vi "纳清叶绿素a电极校准.vi"() -> ()   [LabVIEW 2016, in "斯坦道多参数.lvlib"]
uses:
  <vilib>/Utility/miscctls.llb/LVPointTypeDef.ctl
  <vilib>/Utility/miscctls.llb/LVPositionTypeDef.ctl
  <vilib>/Analysis/NI_AALBase.lvlib
panel:
  in  "量程":u16(ring) items=["0-500", "0-50"]
  out "第三点信号值":dbl
  out "第二点信号值":dbl
  out "第一点信号值":dbl
  out "报警信息":string
  out "通讯状态":string
  out "第三点校准值":dbl
  out "标液3":sgl
  out "第二点校准值":dbl
  out "第一点校准值":dbl
  in  "校准停止":bool
  in  "校准启动":bool
  in  "校准模式":u16(ring)=1 items=["两点校准", "单点校准", "三点校准"]
  out "最小值":sgl format="%#.2f"
  out "最大值":sgl format="%#.2f"
  out "波形图表":dbl(graph) caption="历史曲线"
  out "mean":dbl caption="均值" format="%#.2f"
  out "standard deviation":dbl caption="标准差" format="%#.2f"
  out "变异系数":dbl format="%#.6f"
  out "测量值":sgl format="%#.2f"
  out "提示":string
  out "标液2":sgl
  out "标液1":sgl
  out "原始光强数值":u16 caption="信号值"
  out "温度":dbl format="%#.2f"
  # "叶绿素a电极设定"
  # "℃"
  # "μg/L"
  # "μg/L"
  # "请选择校准模式:"
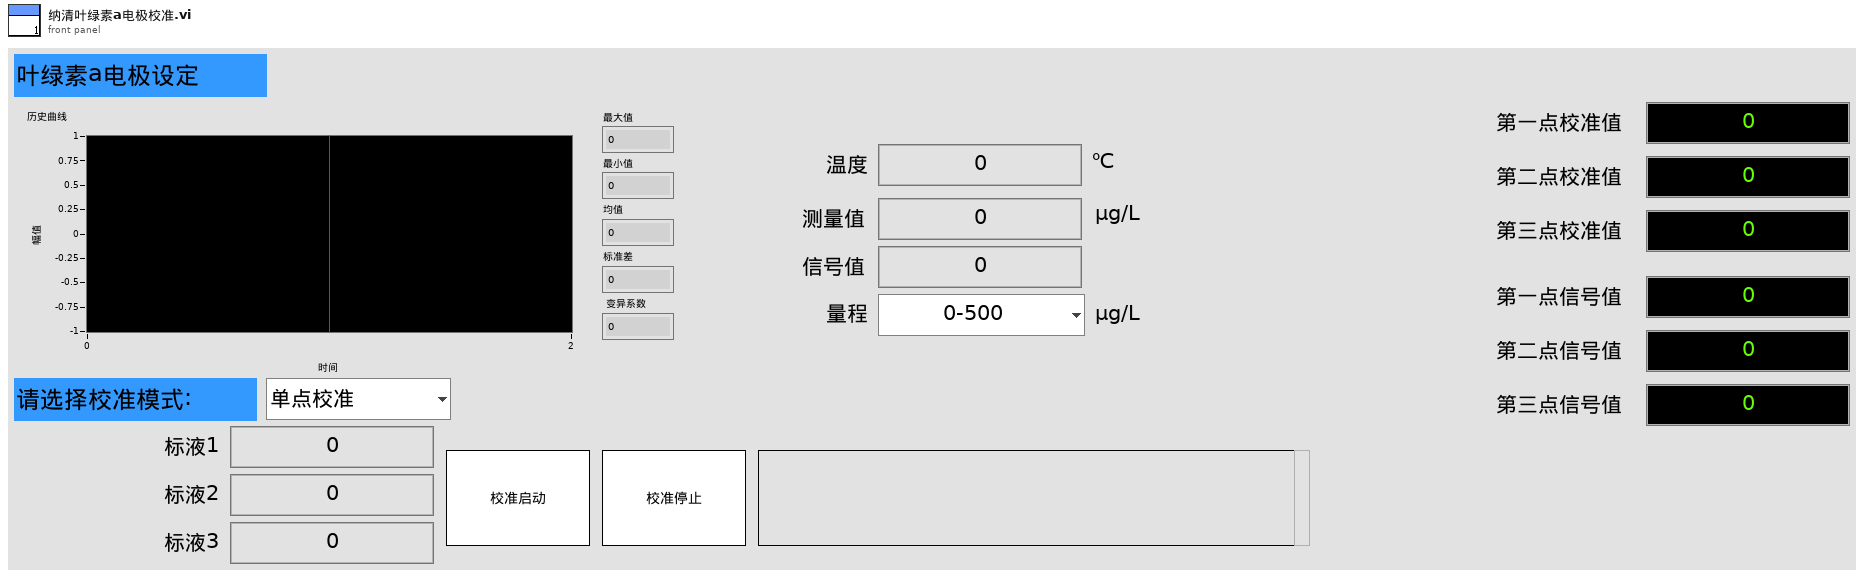
[diagram p1: front panel]
types:
  T1 = typedef "LVPointTypeDef.ctl" = cluster{"Horizontal":i16, "Vertical":i16}
  T2 = cluster{"报警码":u16, "叶绿素a":sgl, "温度数据":sgl, "原始光强数值":u16, "量程":u16, "平均次数":u16, "清扫模式":u16, "清扫次数":u16, "清扫间隔分钟":u16, "0X000B_NC":string, "产品名称":string, "序列号":string, "硬件版本":string, "软件版本":string, "通讯地址":u16, "波特率":u16, "设备类型":u16, "0X0026_NC":string, "校准量程":u16, "第一点原始光强":u16, "第一点校准数据":sgl, "第二点原始光强":u16, "第二点校准数据":sgl, "第三点原始光强":u16, "第三点校准数据":sgl, "探头校准命令":u16, "温度校准参数":sgl, "温度校准命令":u16}
  T3 = typedef "LVPositionTypeDef.ctl" = cluster{"Left":i32, "Top":i32}
  T4 = enum8{"Enabled", "Disabled", "Disabled and Grayed Out"}
  T5 = cluster{"ph":bool, "DO":bool, "Cond":bool, "Turb":bool, "叶绿素a":bool, "藻密度":bool, "ORP":bool}
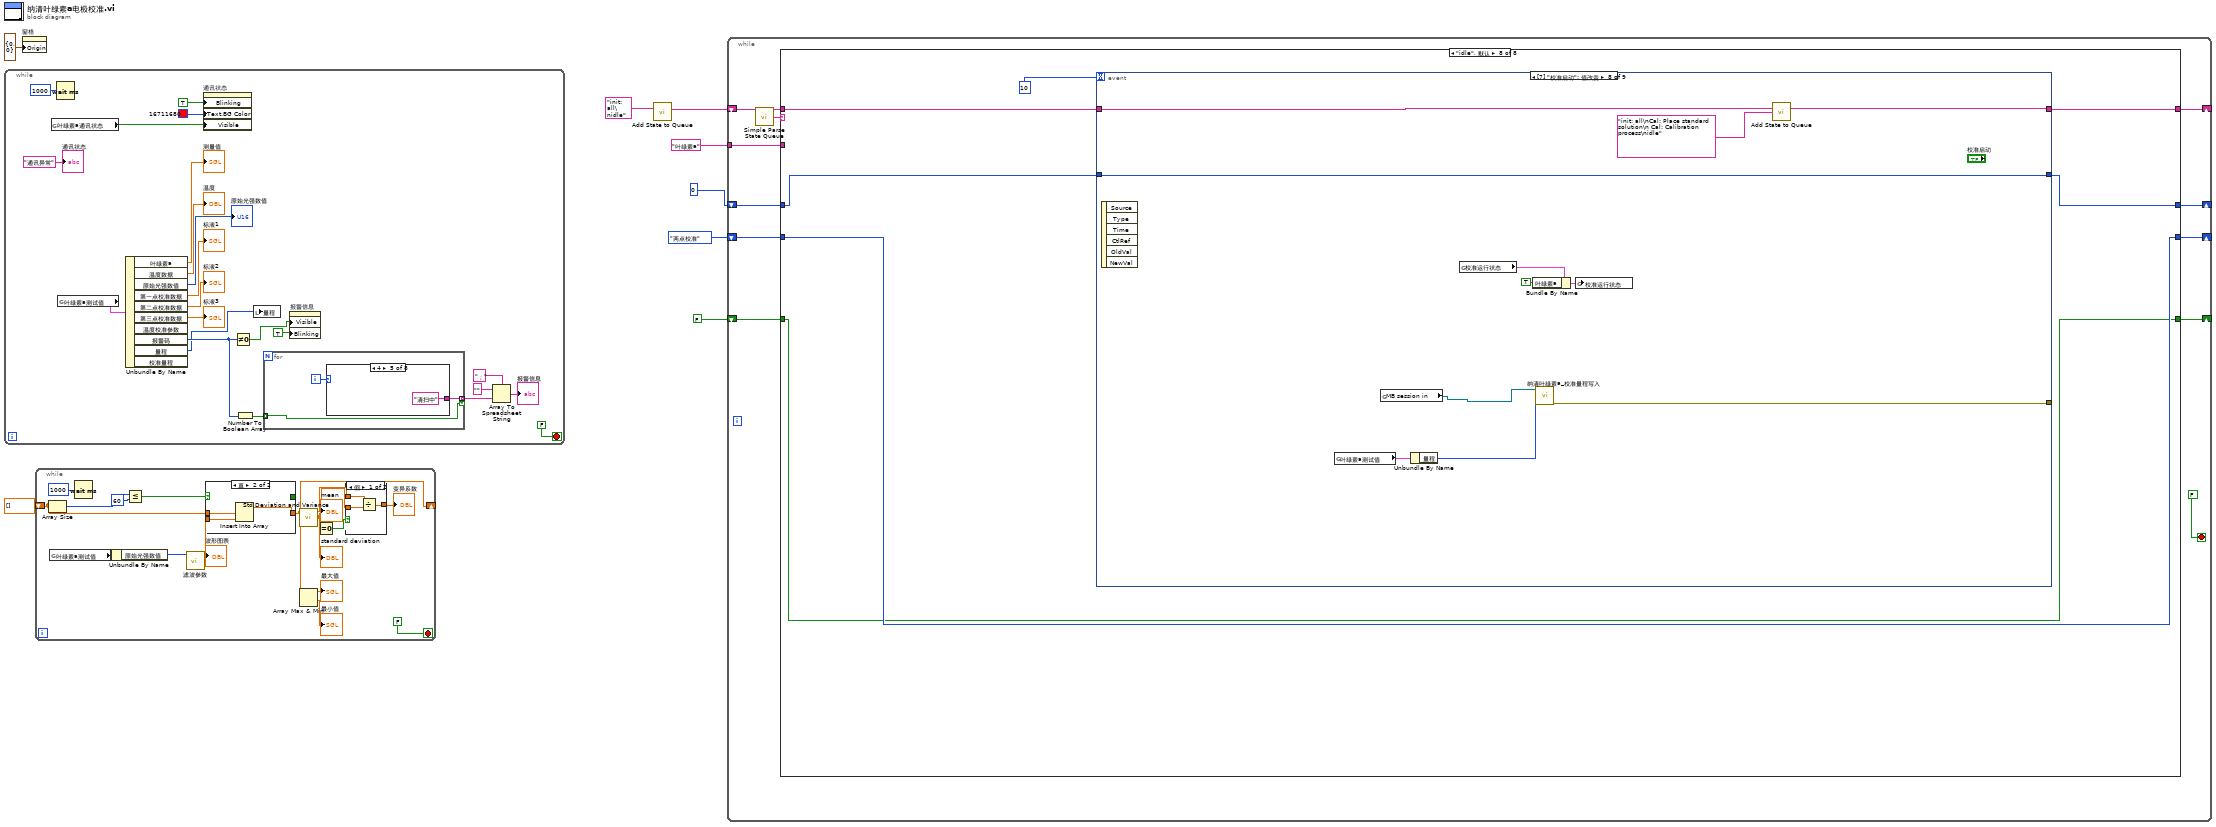
[diagram p0: block diagram]
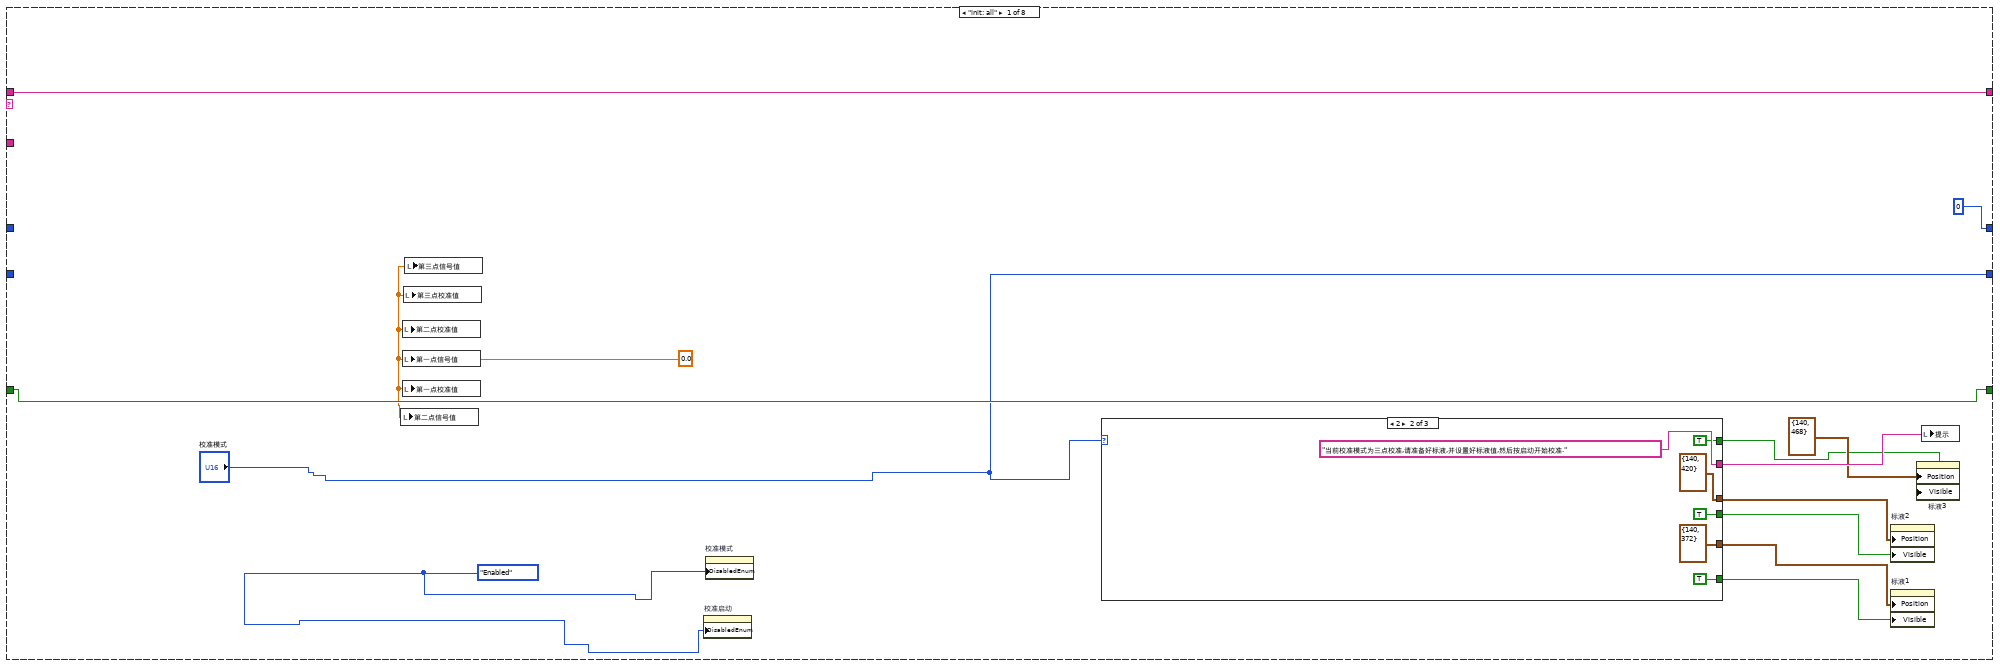
[diagram p2: hidden frame]
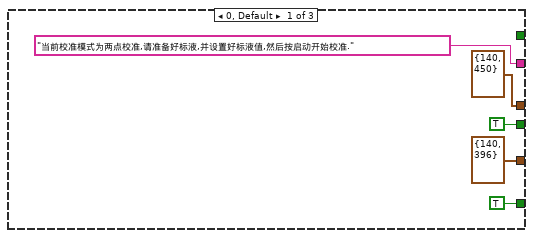
[diagram p3: hidden frame]
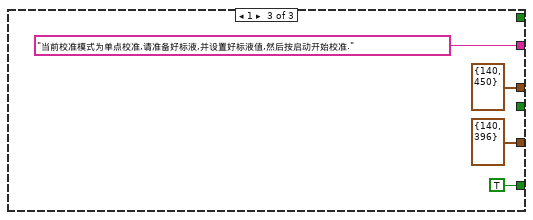
[diagram p4: hidden frame]
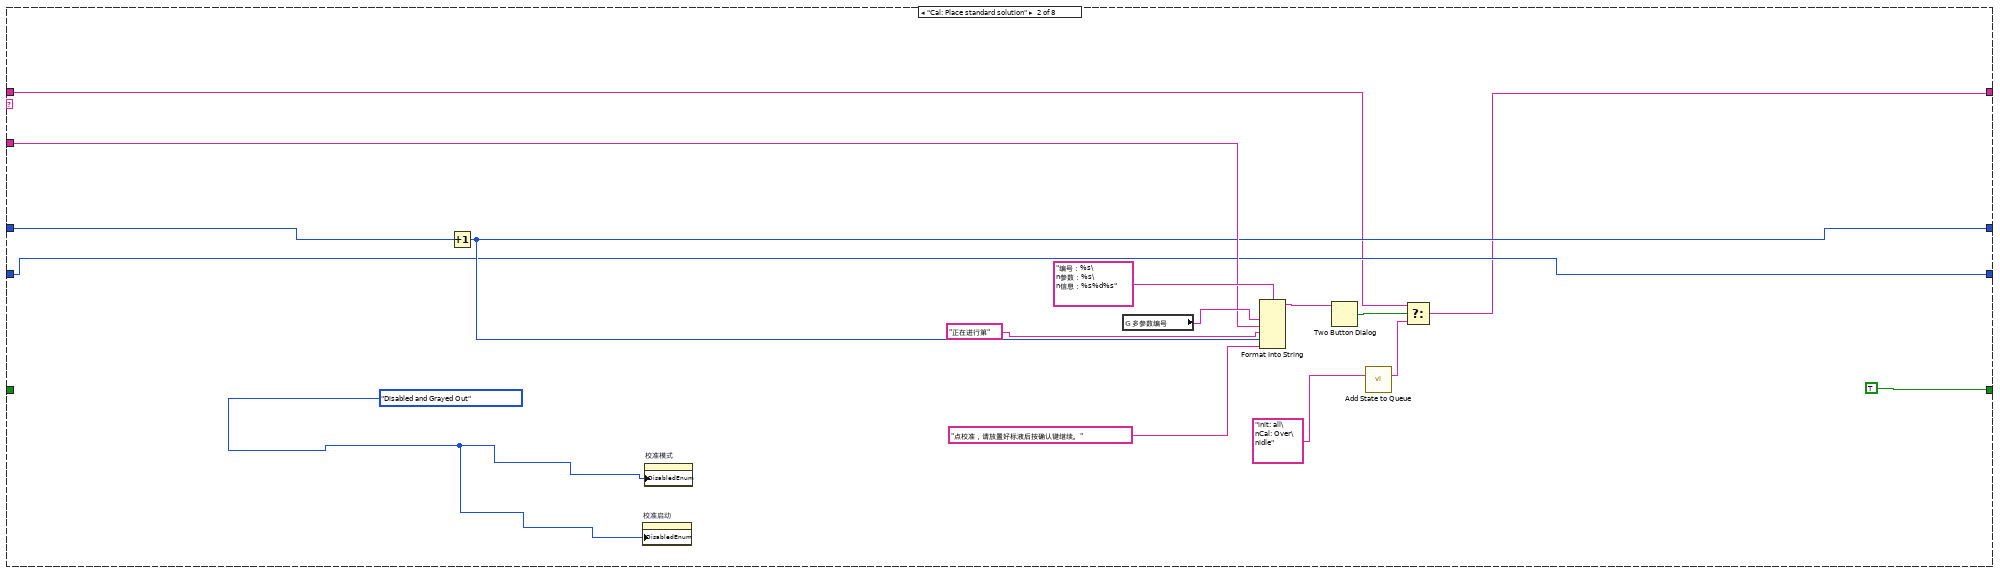
[diagram p5: hidden frame]
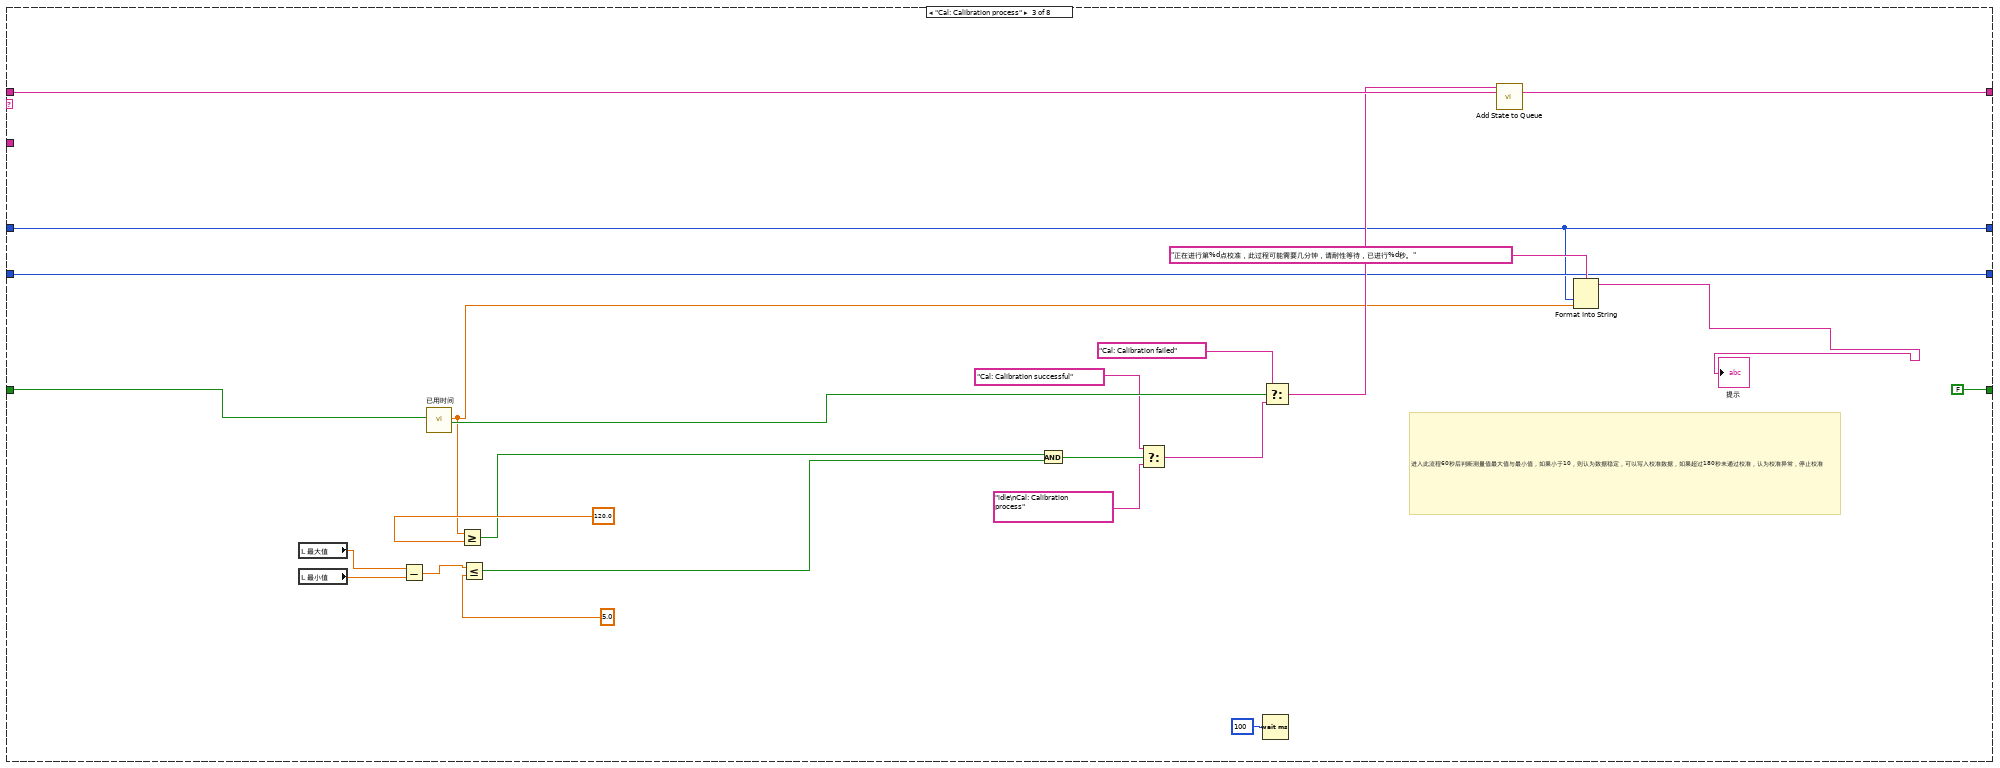
[diagram p6: hidden frame]
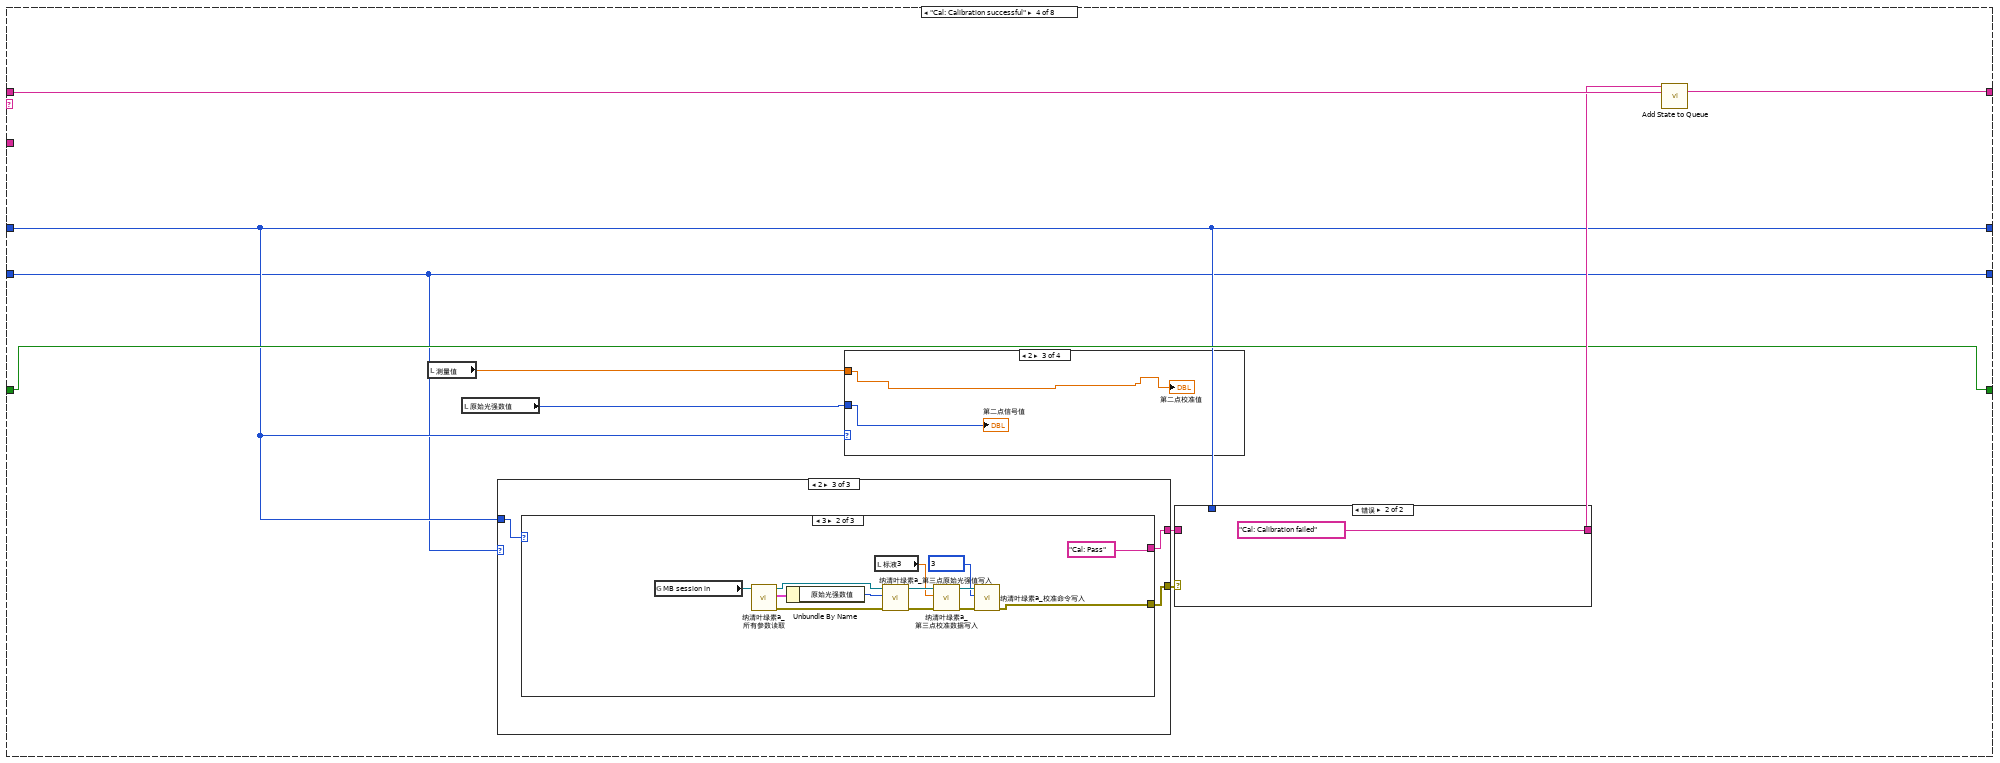
[diagram p7: hidden frame]
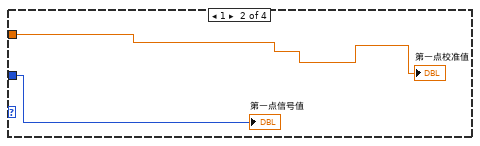
[diagram p9: hidden frame]
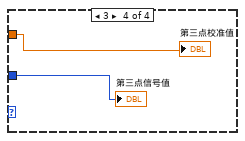
[diagram p10: hidden frame]
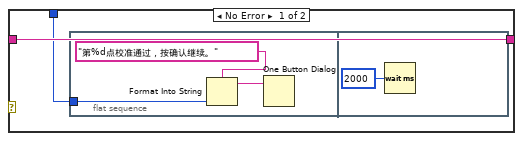
[diagram p11: hidden frame]
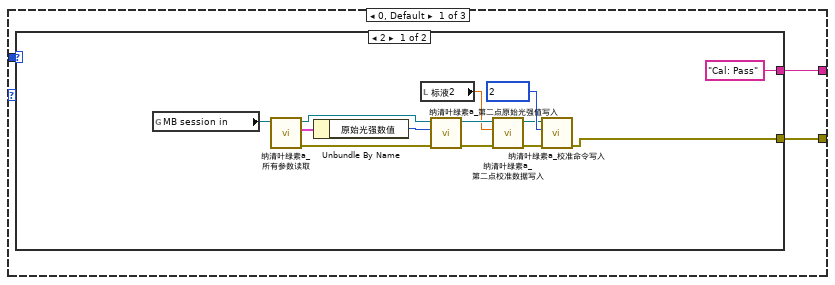
[diagram p12: hidden frame]
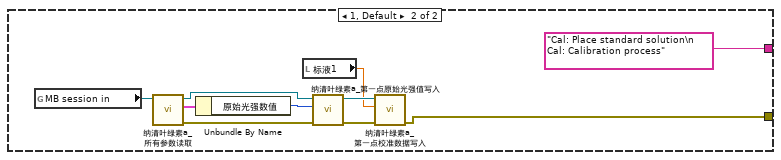
[diagram p13: hidden frame]
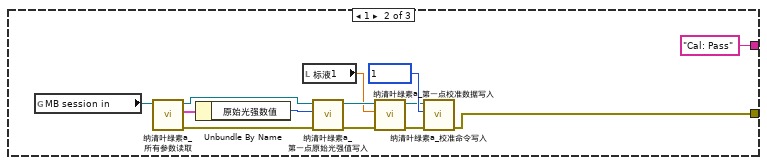
[diagram p14: hidden frame]
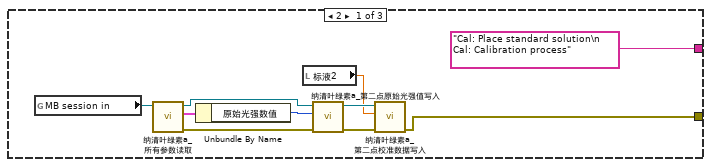
[diagram p15: hidden frame]
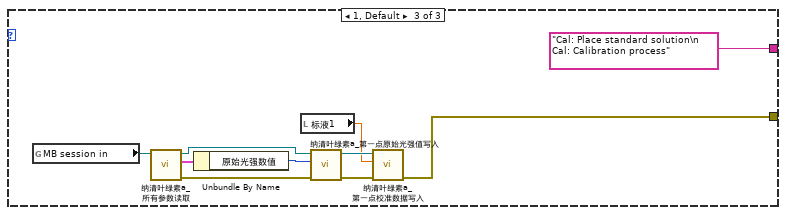
[diagram p16: hidden frame]
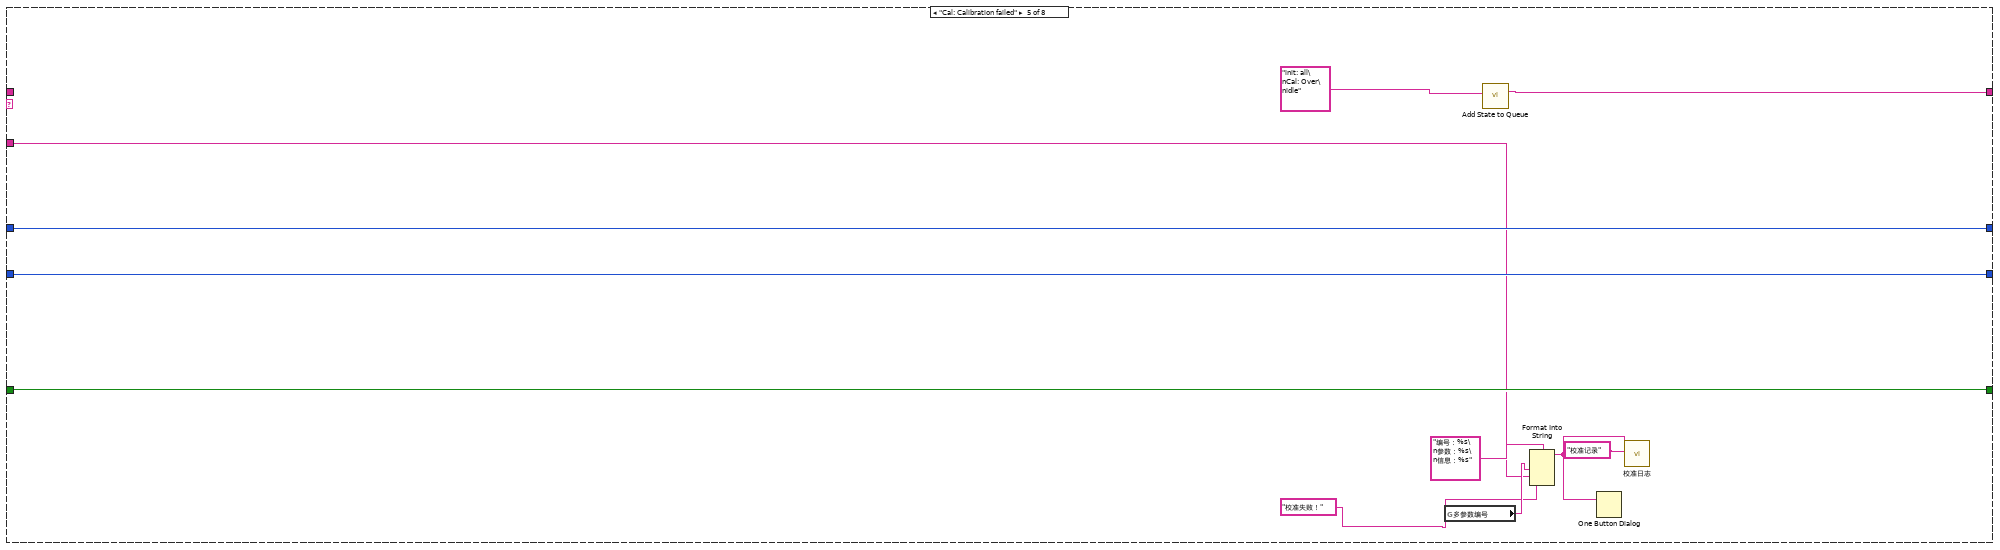
[diagram p17: hidden frame]
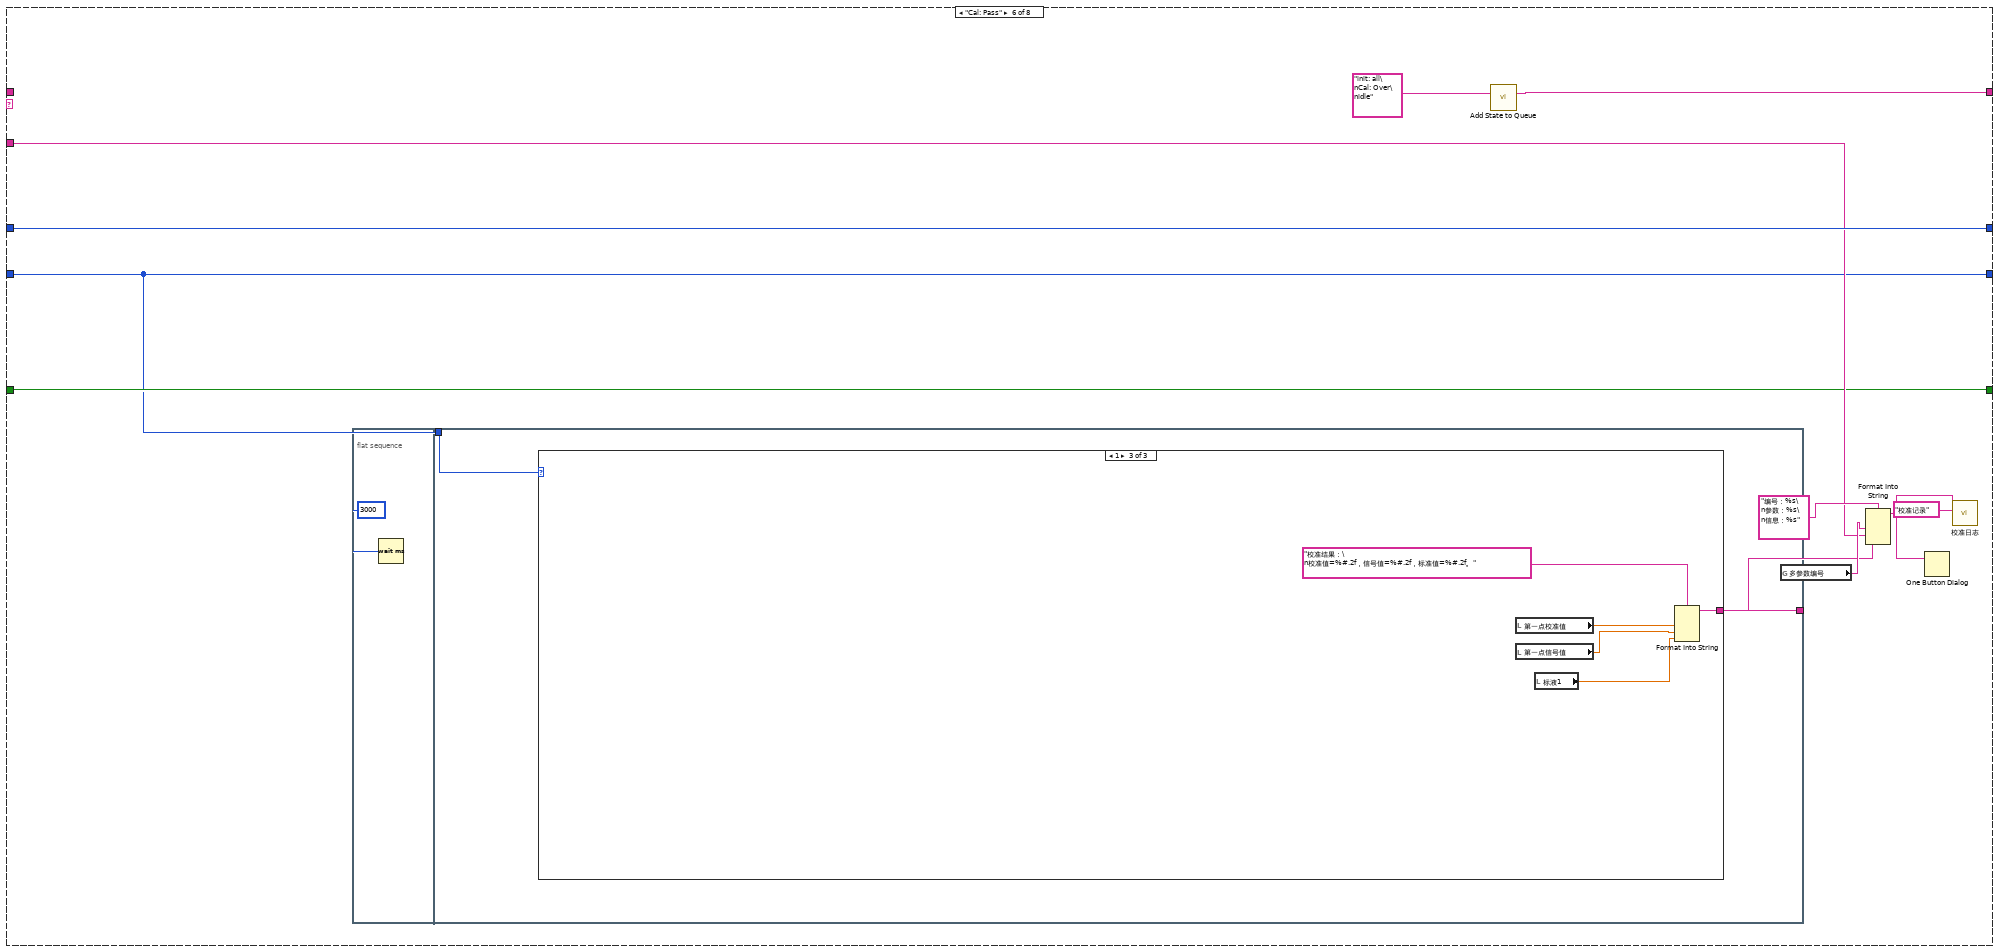
[diagram p18: hidden frame]
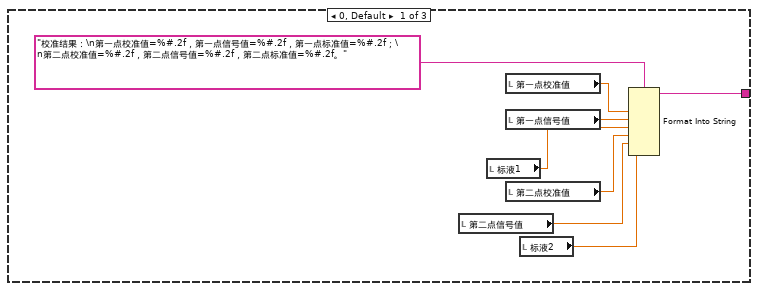
[diagram p19: hidden frame]
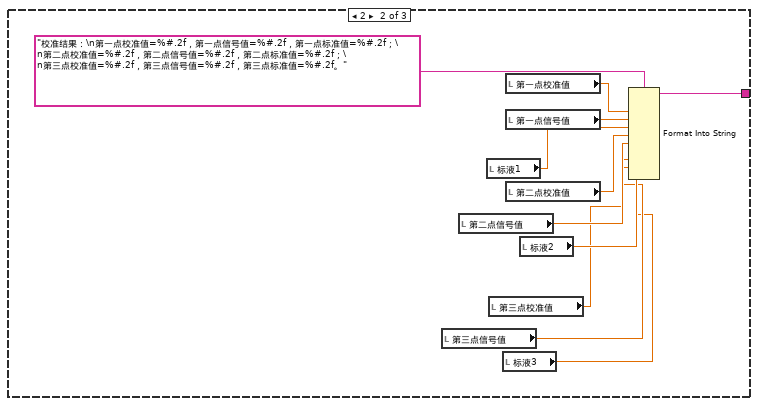
[diagram p20: hidden frame]
diagram:
  n1 = while {
    stop <- FALSE stop-if-true
    n2 = global read "多参数全局变量.vi" "叶绿素a通讯状态"() -> (w18:bool)
    n3 = Wait (ms)(milliseconds to wait=u32 1000 ("等待时间（毫秒）")) -> ()  [unwired: 1 out]
    n4 = global read "纳清过程全局变量.vi" "叶绿素a测试值"() -> (w28:T2)
    n5 = Unbundle By Name(w28) -> ("叶绿素a"=→"测量值":sgl, "温度数据"=→"温度":sgl, "原始光强数值"=→"原始光强数值":u16, "第一点校准数据"=→"标液1":sgl, "第二点校准数据"=→"标液2":sgl, "第三点校准数据"=→"标液3":sgl, "报警码"=w10:u16, "量程"=w9:u16)  [unwired: 2 out]
    n6 = property on="通讯状态" class="Str"("Blinking"=TRUE ("闪烁"), "Text.BG Color"=u32 16711680, "Visible"=w18) -> ()  [unwired: 2 in, 2 out]
    n7 = Not Equal To 0?(x=w10) -> (x != 0?=w12:bool)
    n8 = Number To Boolean Array(number=w10) -> (Boolean array=w17:bool[])
    n9 = local write "量程"(w9) -> ()
    n10 = for {
      tunnel: w17 -> [w31] mode=indexing
      tunnel: [w32] -> w16 mode=indexing if=w31
      i -> [w33]
      n11 = case shown="4" w33 {
        tunnel: [_ "浊度超量程" "温度超量程" "光强信号超范围" "清扫中" "温度传感器故障" "电极故障" "内部电压基准故障"] -> w32
        frame Default {
        }
        frame 0 {
        }
        frame 2 {
        }
        frame 3 {
        }
        frame 4 {
        }
        frame 8 {
        }
        frame 9 {
        }
        frame 10 {
        }
      }
    }
    n12 = property on="报警信息" class="Str"("Visible"=w12, "Blinking"=TRUE ("闪烁")) -> ()  [unwired: 2 in, 2 out]
    n13 = Array To Spreadsheet String(delimiter (Tab)="；" ("分隔符(Tab)"), array=w16, 3:"" ("格式字符串")) -> (spreadsheet string=→"报警信息":string)
    "通讯状态" <- "通讯异常" ("当前串口")
  }
  n14 = property on="窗格" class="Pane"("Origin"=T1 {"Horizontal"=0, "Vertical"=0} ("原点")) -> ()  [unwired: 2 in, 2 out]
  n15 = while {
    shift-right: [w46] -> _
    shift-left: sgl[] [] -> [w52]
    stop <- FALSE stop-if-true
    n16 = Array Size(array=w52) -> (size(s)=w54:i32)
    n17 = global read "纳清过程全局变量.vi" "叶绿素a测试值"() -> (w43:T2)
    n18 = Wait (ms)(milliseconds to wait=u32 1000 ("等待时间（毫秒）")) -> ()  [unwired: 1 out]
    n19 = Unbundle By Name(w43) -> ("原始光强数值"=w42:u16)
    n20 = Less Or Equal?(x=w54, y=60) -> (x <= y?=w53:bool)
    n21 = call "滤波参数.vi"("x"=w42) -> ("mode"=w41:dbl)  [unwired: 10 in]
    "波形图表" <- w41
    n22 = case shown="真" w53 {
      tunnel: w52 -> [w65 w68]
      tunnel: w41 -> [w63 w67]
      tunnel: [w61 w66] -> w46
      tunnel: [TRUE _] -> _
      frame False {
        n23 = Replace Array Subset(array=w65, new element=w63) -> (w64:sgl[])  [unwired: 1 in]
        n24 = Rotate 1D Array(1:w64, 2:-1 ("n")) -> (0:w61:sgl[])
      }
      frame True {
        n25 = Insert Into Array(array=w68, new element=w67) -> (w66:sgl[])  [unwired: 1 in]
      }
    }
    n26 = call <vilib>:"Std Deviation and Variance.vi"("X"=w46) -> ("mean"=w50:dbl, "standard deviation"=w49:dbl)  [unwired: 1 in, 1 out]
    "mean" <- w50
    "standard deviation" <- w49
    n27 = Array Max & Min(array=w46) -> (max value=→"最大值":sgl, min value=→"最小值":sgl)  [unwired: 2 out]
    n28 = Equal To 0?(x=w50) -> (x = 0?=w51:bool)
    n29 = case shown="假" w51 {
      tunnel: w49 -> [w59 _]
      tunnel: [w58 _] -> w48
      tunnel: w50 -> [w57 _]
      frame False {
        n30 = Divide(x=w59, y=w57) -> (x/y=w58:dbl)
      }
      frame True {
      }
    }
    "变异系数" <- w48
  }
  n31 = call "Add State to Queue.vi"("State(s) In (\"\")"="init: all\nidle" ("State(s) In (\"\")")) -> ("States Out"=w5:string)  [unwired: 14 in]
  n32 = while {
    shift-right: [w76] -> _
    shift-left: w5 -> [w80]
    shift-right: [w73] -> _
    shift-left: 0 -> [w75]
    tunnel: "叶绿素a" ("State(s) In (\"\")") -> [w74]
    shift-right: [w71] -> _
    shift-left: enum16{"两点校准", "单点校准", "三点校准"}."两点校准" ("校准模式") -> [w72]
    shift-right: [w69] -> _
    shift-left: FALSE -> [w70]
    stop <- FALSE stop-if-true
    n33 = call "Simple Parse State Queue.vi"("State Queue"=w80) -> ("Remain States"=w77:string, "Next State"=w78:string)  [unwired: 13 in]
    n34 = case shown="\"idle\", 默认" w78 {
      tunnel: w77 -> [w93 w112 w143 w156 _ _ w302 w309]
      tunnel: [w93 w111 w142 w155 w254 w259 w302 w308] -> w76
      tunnel: w75 -> [_ w120 w127 w150 w257 w268 w301 w306]
      tunnel: w74 -> [_ w121 _ _ w248 w264 _ _]
      tunnel: [0 w118 w127 w150 w257 w268 w301 w307] -> w73
      tunnel: w72 -> [_ w117 w128 w149 w256 w260 w300 w305]
      tunnel: ["校准模式" w117 w128 w149 w256 w260 w300 w305] -> w71
      tunnel: w70 -> [w91 _ w130 w151 w255 w263 w299 w303]
      tunnel: [w91 TRUE FALSE w151 w255 w263 w299 w303] -> w69
      frame "init: all" {
        w88 = T4."Enabled" ("禁用")
        w90 = 0.0 ("第一点校准值")
        n35 = local write "第二点信号值"(w90) -> ()
        n36 = local write "第二点校准值"(w90) -> ()
        n37 = local write "第一点信号值"(w90) -> ()
        n38 = local write "第一点校准值"(w90) -> ()
        n39 = local write "第三点校准值"(w90) -> ()
        n40 = local write "第三点信号值"(w90) -> ()
        n41 = property on="校准启动" class="Bool"("DisabledEnum"=w88) -> ()  [unwired: 2 in, 2 out]
        n42 = property on="校准模式" class="Ring (严格)"("DisabledEnum"=w88) -> ()  [unwired: 2 in, 2 out]
        n43 = case shown="2" "校准模式" {
          tunnel: ["当前校准模式为两点校准,请准备好标液,并设置好标液值,然后按启动开始校准." ("提示") "当前校准模式为三点校准,请准备好标液,并设置好标液值,然后按启动开始校准." ("提示") "当前校准模式为单点校准,请准备好标液,并设置好标液值,然后按启动开始校准." ("提示")] -> w89
          tunnel: [TRUE ("可见") TRUE ("可见") _] -> w83
          tunnel: [T3 {"Left"=140, "Top"=396} ("位置") T3 {"Left"=140, "Top"=372} ("位置") T3 {"Left"=140, "Top"=396} ("位置")] -> w82
          tunnel: [T3 {"Left"=140, "Top"=450} ("位置 2") T3 {"Left"=140, "Top"=420} ("位置 2") T3 {"Left"=140, "Top"=450} ("位置 2")] -> w84
          tunnel: [_ TRUE ("可见") _] -> w85
          tunnel: [TRUE ("可见") TRUE ("可见") TRUE ("可见")] -> w81
          frame 0, Default {
          }
          frame 2 {
          }
          frame 1 {
          }
        }
        n44 = property on="标液2" class="DigNum (严格)"("Position"=w84, "Visible"=w83) -> ()  [unwired: 2 in, 2 out]
        n45 = property on="标液1" class="DigNum (严格)"("Position"=w82, "Visible"=w81) -> ()  [unwired: 2 in, 2 out]
        n46 = property on="标液3" class="DigNum (严格)"("Position"=T3 {"Left"=140, "Top"=468} ("位置 3"), "Visible"=w85) -> ()  [unwired: 2 in, 2 out]
        n47 = local write "提示"(w89) -> ()
      }
      frame "Cal: Place standard solution" {
        w110 = T4."Disabled and Grayed Out" ("禁用")
        n48 = Increment(x=w120) -> (x+1=w118:i32)
        n49 = property on="校准启动" class="Bool"("DisabledEnum"=w110) -> ()  [unwired: 2 in, 2 out]
        n50 = property on="校准模式" class="Ring (严格)"("DisabledEnum"=w110) -> ()  [unwired: 2 in, 2 out]
        n51 = global read "多参数全局变量.vi" "多参数编号"() -> (w123:string)
        n52 = Format Into String(format string="编号：%s\n参数：%s\n信息：%s%d%s" ("格式字符串"), w123, w121, "正在进行第" ("消息"), w118, "点校准，请放置好标液后按确认键继续。" ("消息")) -> (resulting string=w115:string)  [unwired: 2 in, 1 out]
        n53 = Two Button Dialog(message=w115) -> (T button?=w114:bool)  [unwired: 2 in]
        n54 = call "Add State to Queue.vi"("State(s) In (\"\")"="init: all\nCal: Over\nidle" ("State(s) In (\"\")")) -> ("States Out"=w113:string)  [unwired: 14 in]
        n55 = Select(t=w112, s=w114, f=w113) -> (s? t:f=w111:string)
      }
      frame "Cal: Calibration process" {
        # "进入此流程60秒后判断测量值最大值与最小值，如果小于10，则认为数据稳定，可以写入校准数据，如果超过180秒未通过校准，认为校准异常，停止校准"
        n56 = local read "最大值"() -> (w147:sgl)
        n57 = local read "最小值"() -> (w146:sgl)
        n58 = Subtract(x=w147, y=w146) -> (x-y=w148:sgl)
        n59 = call "已用时间"("Reset"=w130) -> ("Elapsed Time (s)"=w126:dbl, "Time has Elapsed"=w144:bool)  [unwired: 11 in, 6 out]
        n60 = Greater Or Equal?(x=w126, y=120.0) -> (x >= y?=w139:bool)
        n61 = Less Or Equal?(x=w148, y=5.0) -> (x <= y?=w135:bool)
        n62 = And(x=w139, y=w135) -> (x .and. y?=w136:bool)
        n63 = Select(t="Cal: Calibration successful" ("State(s) In (\"\")"), s=w136, f="idle\nCal: Calibration process" ("State(s) In (\"\")")) -> (s? t:f=w134:string)
        n64 = Wait (ms)(milliseconds to wait=u32 100 ("等待时间（毫秒）")) -> ()  [unwired: 1 out]
        n65 = Select(t="Cal: Calibration failed" ("State(s) In (\"\")"), s=w144, f=w134) -> (s? t:f=w133:string)
        n66 = call "Add State to Queue.vi"("State(s) In Front (\"\")"=w133, "State(s) In (\"\")"=w143) -> ("States Out"=w142:string)  [unwired: 13 in]
        n67 = Format Into String(format string="正在进行第%d点校准，此过程可能需要几分钟，请耐性等待，已进行%d秒。" ("格式字符串"), w127, w126) -> (resulting string=→"提示":string)  [unwired: 2 in, 1 out]
      }
      frame "Cal: Calibration successful" {
        n68 = local read "测量值"() -> (w152:sgl)
        n69 = local read "原始光强数值"() -> (w153:u16)
        n70 = case shown="2" w149 {
          tunnel: [w174 w198 w211] -> w158
          tunnel: [w173 "Cal: Pass" ("State(s) In (\"\")") w212] -> w157
          tunnel: w150 -> [w172 _ w213]
          frame 0, Default {
            n71 = case shown="2" w172 {
              tunnel: [w175 w188] -> w174
              tunnel: ["Cal: Pass" ("State(s) In (\"\")") "Cal: Place standard solution\n Cal: Calibration process" ("State(s) In (\"\")")] -> w173
              frame 2 {
                n72 = global read "多参数全局变量.vi" "MB session in"() -> (w183:refnum<class "MB_Master.lvclass">)
                n73 = call "纳清叶绿素a_所有参数读取.vi"("MB session in"=w183) -> ("error out"=w185:errorcluster, "输出值"=w182:T2, "MB session out"=w184:refnum<class "MB_Master.lvclass">)  [unwired: 8 in]
                n74 = Unbundle By Name(w182) -> ("原始光强数值"=w181:u16)
                n75 = local read "标液2"() -> (w176:sgl)
                n76 = call "纳清叶绿素a_第二点原始光强值写入.vi"("error in (no error)"=w185, "数值"=w181, "MB session in"=w184) -> ("error out"=w180:errorcluster, "MB session out"=w179:refnum<class "MB_Master.lvclass">)  [unwired: 7 in]
                n77 = call "纳清叶绿素a_第二点校准数据写入.vi"("error in (no error)"=w180, "数值"=w176, "MB session in"=w179) -> ("error out"=w178:errorcluster, "MB session out"=w177:refnum<class "MB_Master.lvclass">)  [unwired: 7 in]
                n78 = call "纳清叶绿素a_校准命令写入.vi"("error in (no error)"=w178, "数值"=u16 2 ("starting address"), "MB session in"=w177) -> ("error out"=w175:errorcluster)  [unwired: 7 in, 1 out]
              }
              frame 1, Default {
                n79 = global read "多参数全局变量.vi" "MB session in"() -> (w194:refnum<class "MB_Master.lvclass">)
                n80 = call "纳清叶绿素a_所有参数读取.vi"("MB session in"=w194) -> ("error out"=w196:errorcluster, "输出值"=w193:T2, "MB session out"=w195:refnum<class "MB_Master.lvclass">)  [unwired: 8 in]
                n81 = Unbundle By Name(w193) -> ("原始光强数值"=w192:u16)
                n82 = local read "标液1"() -> (w189:sgl)
                n83 = call "纳清叶绿素a_第一点原始光强值写入.vi"("error in (no error)"=w196, "数值"=w192, "MB session in"=w195) -> ("error out"=w191:errorcluster, "MB session out"=w190:refnum<class "MB_Master.lvclass">)  [unwired: 7 in]
                n84 = call "纳清叶绿素a_第一点校准数据写入.vi"("error in (no error)"=w191, "数值"=w189, "MB session in"=w190) -> ("error out"=w188:errorcluster)  [unwired: 7 in, 1 out]
              }
            }
          }
          frame 1 {
            n85 = global read "多参数全局变量.vi" "MB session in"() -> (w206:refnum<class "MB_Master.lvclass">)
            n86 = call "纳清叶绿素a_所有参数读取.vi"("MB session in"=w206) -> ("error out"=w208:errorcluster, "输出值"=w205:T2, "MB session out"=w207:refnum<class "MB_Master.lvclass">)  [unwired: 8 in]
            n87 = Unbundle By Name(w205) -> ("原始光强数值"=w204:u16)
            n88 = local read "标液1"() -> (w199:sgl)
            n89 = call "纳清叶绿素a_第一点原始光强值写入.vi"("error in (no error)"=w208, "数值"=w204, "MB session in"=w207) -> ("error out"=w203:errorcluster, "MB session out"=w202:refnum<class "MB_Master.lvclass">)  [unwired: 7 in]
            n90 = call "纳清叶绿素a_第一点校准数据写入.vi"("error in (no error)"=w203, "数值"=w199, "MB session in"=w202) -> ("error out"=w201:errorcluster, "MB session out"=w200:refnum<class "MB_Master.lvclass">)  [unwired: 7 in]
            n91 = call "纳清叶绿素a_校准命令写入.vi"("error in (no error)"=w201, "数值"=u16 1 ("starting address"), "MB session in"=w200) -> ("error out"=w198:errorcluster)  [unwired: 7 in, 1 out]
          }
          frame 2 {
            n92 = case shown="3" w213 {
              tunnel: [w214 w224 w237] -> w211
              tunnel: ["Cal: Place standard solution\n Cal: Calibration process" ("State(s) In (\"\")") "Cal: Pass" ("State(s) In (\"\")") "Cal: Place standard solution\n Cal: Calibration process" ("State(s) In (\"\")")] -> w212
              frame 2 {
                n93 = global read "多参数全局变量.vi" "MB session in"() -> (w220:refnum<class "MB_Master.lvclass">)
                n94 = call "纳清叶绿素a_所有参数读取.vi"("MB session in"=w220) -> ("error out"=w222:errorcluster, "输出值"=w219:T2, "MB session out"=w221:refnum<class "MB_Master.lvclass">)  [unwired: 8 in]
                n95 = Unbundle By Name(w219) -> ("原始光强数值"=w218:u16)
                n96 = local read "标液2"() -> (w215:sgl)
                n97 = call "纳清叶绿素a_第二点原始光强值写入.vi"("error in (no error)"=w222, "数值"=w218, "MB session in"=w221) -> ("error out"=w217:errorcluster, "MB session out"=w216:refnum<class "MB_Master.lvclass">)  [unwired: 7 in]
                n98 = call "纳清叶绿素a_第二点校准数据写入.vi"("error in (no error)"=w217, "数值"=w215, "MB session in"=w216) -> ("error out"=w214:errorcluster)  [unwired: 7 in, 1 out]
              }
              frame 3 {
                n99 = global read "多参数全局变量.vi" "MB session in"() -> (w233:refnum<class "MB_Master.lvclass">)
                n100 = call "纳清叶绿素a_所有参数读取.vi"("MB session in"=w233) -> ("error out"=w235:errorcluster, "输出值"=w232:T2, "MB session out"=w234:refnum<class "MB_Master.lvclass">)  [unwired: 8 in]
                n101 = Unbundle By Name(w232) -> ("原始光强数值"=w231:u16)
                n102 = local read "标液3"() -> (w225:sgl)
                n103 = call "纳清叶绿素a_第三点原始光强值写入.vi"("error in (no error)"=w235, "数值"=w231, "MB session in"=w234) -> ("error out"=w230:errorcluster, "MB session out"=w229:refnum<class "MB_Master.lvclass">)  [unwired: 7 in]
                n104 = call "纳清叶绿素a_第三点校准数据写入.vi"("error in (no error)"=w230, "数值"=w225, "MB session in"=w229) -> ("error out"=w228:errorcluster, "MB session out"=w227:refnum<class "MB_Master.lvclass">)  [unwired: 7 in]
                n105 = call "纳清叶绿素a_校准命令写入.vi"("error in (no error)"=w228, "数值"=u16 3 ("starting address"), "MB session in"=w227) -> ("error out"=w224:errorcluster)  [unwired: 7 in, 1 out]
              }
              frame 1, Default {
                n106 = global read "多参数全局变量.vi" "MB session in"() -> (w243:refnum<class "MB_Master.lvclass">)
                n107 = call "纳清叶绿素a_所有参数读取.vi"("MB session in"=w243) -> ("error out"=w245:errorcluster, "输出值"=w242:T2, "MB session out"=w244:refnum<class "MB_Master.lvclass">)  [unwired: 8 in]
                n108 = Unbundle By Name(w242) -> ("原始光强数值"=w241:u16)
                n109 = local read "标液1"() -> (w238:sgl)
                n110 = call "纳清叶绿素a_第一点原始光强值写入.vi"("error in (no error)"=w245, "数值"=w241, "MB session in"=w244) -> ("error out"=w240:errorcluster, "MB session out"=w239:refnum<class "MB_Master.lvclass">)  [unwired: 7 in]
                n111 = call "纳清叶绿素a_第一点校准数据写入.vi"("error in (no error)"=w240, "数值"=w238, "MB session in"=w239) -> ("error out"=w237:errorcluster)  [unwired: 7 in, 1 out]
              }
            }
          }
        }
        n112 = case shown="2" w150 {
          tunnel: w153 -> [_ w160 w162 w164]
          tunnel: w152 -> [_ w159 w161 w163]
          frame 0, Default {
          }
          frame 1 {
            "第一点信号值" <- w160
            "第一点校准值" <- w159
          }
          frame 2 {
            "第二点信号值" <- w162
            "第二点校准值" <- w161
          }
          frame 3 {
            "第三点信号值" <- w164
            "第三点校准值" <- w163
          }
        }
        n113 = case shown="错误" w158 {
          tunnel: w157 -> [w166 _]
          tunnel: [w166 "Cal: Calibration failed" ("State(s) In (\"\")")] -> w154
          tunnel: w150 -> [w165 _]
          frame No Error {
            n114 = flat-sequence {
              tunnel: w165 -> [w167]
              frame #0 {
                n115 = Format Into String(format string="第%d点校准通过，按确认继续。" ("格式字符串"), w167) -> (resulting string=w169:string)  [unwired: 2 in, 1 out]
                n116 = One Button Dialog(message=w169) -> ()  [unwired: 1 in, 1 out]
              }
              frame #1 {
                n117 = Wait (ms)(milliseconds to wait=u32 2000 ("等待时间（毫秒）")) -> ()  [unwired: 1 out]
              }
            }
          }
          frame Error {
          }
        }
        n118 = call "Add State to Queue.vi"("State(s) In Front (\"\")"=w154, "State(s) In (\"\")"=w156) -> ("States Out"=w155:string)  [unwired: 13 in]
      }
      frame "Cal: Calibration failed" {
        n119 = global read "多参数全局变量.vi" "多参数编号"() -> (w251:string)
        n120 = call "Add State to Queue.vi"("State(s) In (\"\")"="init: all\nCal: Over\nidle" ("State(s) In (\"\")")) -> ("States Out"=w254:string)  [unwired: 14 in]
        n121 = Format Into String(format string="编号：%s\n参数：%s\n信息：%s" ("格式字符串"), w251, w248, "校准失败！" ("消息")) -> (resulting string=w250:string)  [unwired: 2 in, 1 out]
        n122 = One Button Dialog(message=w250) -> ()  [unwired: 1 in, 1 out]
        n123 = call "校准日志.vi"("table"="校准记录", "日志信息"=w250) -> ()  [unwired: 9 in, 1 out]
      }
      frame "Cal: Pass" {
        n124 = flat-sequence {
          tunnel: [w271] -> w261
          tunnel: w260 -> [w270]
          frame #0 {
            n125 = Wait (ms)(milliseconds to wait=u32 3000 ("等待时间（毫秒）")) -> ()  [unwired: 1 out]
          }
          frame #1 {
            n126 = case shown="1" w270 {
              tunnel: [w279 w290 w295] -> w271
              frame 0, Default {
                n127 = local read "第二点信号值"() -> (w273:dbl)
                n128 = local read "标液1"() -> (w275:sgl)
                n129 = local read "第一点校准值"() -> (w277:dbl)
                n130 = local read "第一点信号值"() -> (w278:dbl)
                n131 = local read "第二点校准值"() -> (w274:dbl)
                n132 = local read "标液2"() -> (w272:sgl)
                n133 = Format Into String(format string="校准结果：\n第一点校准值=%#.2f，第一点信号值=%#.2f，第一点标准值=%#.2f；\n第二点校准值=%#.2f，第二点信号值=%#.2f，第二点标准值=%#.2f。" ("提示"), w277, w278, w275, w274, w273, w272) -> (resulting string=w279:string)  [unwired: 2 in, 1 out]
              }
              frame 2 {
                n134 = local read "第三点信号值"() -> (w281:dbl)
                n135 = local read "第二点信号值"() -> (w284:dbl)
                n136 = local read "标液1"() -> (w286:sgl)
                n137 = local read "第三点校准值"() -> (w282:dbl)
                n138 = local read "标液3"() -> (w280:sgl)
                n139 = local read "第一点校准值"() -> (w288:dbl)
                n140 = local read "第一点信号值"() -> (w289:dbl)
                n141 = local read "第二点校准值"() -> (w285:dbl)
                n142 = local read "标液2"() -> (w283:sgl)
                n143 = Format Into String(format string="校准结果：\n第一点校准值=%#.2f，第一点信号值=%#.2f，第一点标准值=%#.2f；\n第二点校准值=%#.2f，第二点信号值=%#.2f，第二点标准值=%#.2f；\n第三点校准值=%#.2f，第三点信号值=%#.2f，第三点标准值=%#.2f。" ("提示"), w288, w289, w286, w285, w284, w283, w282, w281, w280) -> (resulting string=w290:string)  [unwired: 2 in, 1 out]
              }
              frame 1 {
                n144 = local read "第一点校准值"() -> (w294:dbl)
                n145 = local read "第一点信号值"() -> (w292:dbl)
                n146 = local read "标液1"() -> (w291:sgl)
                n147 = Format Into String(format string="校准结果：\n校准值=%#.2f，信号值=%#.2f，标准值=%#.2f。" ("提示"), w294, w292, w291) -> (resulting string=w295:string)  [unwired: 2 in, 1 out]
              }
            }
          }
        }
        n148 = call "Add State to Queue.vi"("State(s) In (\"\")"="init: all\nCal: Over\nidle" ("State(s) In (\"\")")) -> ("States Out"=w259:string)  [unwired: 14 in]
        n149 = global read "多参数全局变量.vi" "多参数编号"() -> (w265:string)
        n150 = Format Into String(format string="编号：%s\n参数：%s\n信息：%s" ("格式字符串"), w265, w264, w261) -> (resulting string=w262:string)  [unwired: 2 in, 1 out]
        n151 = One Button Dialog(message=w262) -> ()  [unwired: 1 in, 1 out]
        n152 = call "校准日志.vi"("table"="校准记录", "日志信息"=w262) -> ()  [unwired: 9 in, 1 out]
      }
      frame "Cal: Over" {
        n153 = global read "多参数全局变量.vi" "校准运行状态"() -> (w297:T5)
        n154 = Bundle By Name(cluster=w297, "叶绿素a"=FALSE ("Cond")) -> (w298:T5)
        n155 = global write "多参数全局变量.vi" "校准运行状态"(w298) -> ()
      }
      frame "idle", Default {
        n156 = event shown="[7] \"校准启动\": 值改变" {
          selector: _ -> [_ _ _ _ _ _ _ _ _]
          dyn-events: _ -> [_ _ _ _ _ _ _ _ _]
          timeout: 10 -> [_ _ _ _ _ _ _ _ _]
          tunnel: w309 -> [w312 w316 w319 w326 w331 w336 w343 w356 _]
          tunnel: [w311 w315 w320 w330 w335 w340 w345 w355 w358] -> w308
          tunnel: [w310 w313 w321 w329 w334 w339 w344 w353 w359] -> w307
          tunnel: w306 -> [w310 w313 w321 w329 w334 w339 w344 w353 w359]
          tunnel: [_ _ _ _ _ _ _ w346 _] -> _
          event Timeout {
            n157 = event-data() -> ()  [unwired: 1 in, 3 out]
            n158 = call "Add State to Queue.vi"("State(s) In (\"\")"=w312) -> ("States Out"=w311:string)  [unwired: 14 in]
          }
          event "校准模式": Value Change {
            n159 = event-data() -> ()  [unwired: 1 in, 6 out]
            n160 = call "Add State to Queue.vi"("State(s) In (\"\")"=w316, "State(s) At Back (\"\")"="init: all\nidle" ("State(s) In (\"\")")) -> ("States Out"=w315:string)  [unwired: 13 in]
          }
          event "标液1", "标液2", "标液3": Mouse Down {
            n161 = event-data() -> ("CtlRef"=w318:refnum<vi>)  [unwired: 1 in, 7 out]
            n162 = property class="DigNum (严格)"(reference=w318) -> ("DisabledEnum"=w317:T4)  [unwired: 1 in, 2 out]
            n163 = case shown="\"Enabled\"" w317 {
              tunnel: w318 -> [w325 _]
              frame "Enabled" {
                n164 = property class="DigNum (严格)"(reference=w325) -> (reference out=w322:refnum<vi>, "Value"=w323:sgl)  [unwired: 1 in, 1 out]
                n165 = call "数字键盘.vi"("OldNumber"=w323) -> ("NewNumber"=w324:dbl)  [unwired: 1 in]
                n166 = property class="DigNum (严格)"(reference=w322, "Val(Sgnl)"=w324) -> ()  [unwired: 1 in, 2 out]
              }
              frame "Disabled", Default {
              }
            }
            n167 = call "Add State to Queue.vi"("State(s) In (\"\")"=w319) -> ("States Out"=w320:string)  [unwired: 14 in]
          }
          event "标液1": Value Change {
            n168 = event-data() -> ("NewVal"=w327:sgl)  [unwired: 1 in, 5 out]
            n169 = global read "多参数全局变量.vi" "MB session in"() -> (w328:refnum<class "MB_Master.lvclass">)
            n170 = call "纳清叶绿素a_第一点校准数据写入.vi"("数值"=w327, "MB session in"=w328) -> ()  [unwired: 8 in, 2 out]
            n171 = call "Add State to Queue.vi"("State(s) In (\"\")"=w326) -> ("States Out"=w330:string)  [unwired: 14 in]
          }
          event "标液2": Value Change {
            n172 = event-data() -> ("NewVal"=w332:sgl)  [unwired: 1 in, 5 out]
            n173 = global read "多参数全局变量.vi" "MB session in"() -> (w333:refnum<class "MB_Master.lvclass">)
            n174 = call "纳清叶绿素a_第二点校准数据写入.vi"("数值"=w332, "MB session in"=w333) -> ()  [unwired: 8 in, 2 out]
            n175 = call "Add State to Queue.vi"("State(s) In (\"\")"=w331) -> ("States Out"=w335:string)  [unwired: 14 in]
          }
          event "标液3": Value Change {
            n176 = event-data() -> ("NewVal"=w337:sgl)  [unwired: 1 in, 5 out]
            n177 = global read "多参数全局变量.vi" "MB session in"() -> (w338:refnum<class "MB_Master.lvclass">)
            n178 = call "纳清叶绿素a_第三点校准数据写入.vi"("数值"=w337, "MB session in"=w338) -> ()  [unwired: 8 in, 2 out]
            n179 = call "Add State to Queue.vi"("State(s) In (\"\")"=w336) -> ("States Out"=w340:string)  [unwired: 14 in]
          }
          event "量程": Value Change {
            n180 = event-data() -> ("NewVal"=w341:u16)  [unwired: 1 in, 5 out]
            n181 = global read "多参数全局变量.vi" "MB session in"() -> (w342:refnum<class "MB_Master.lvclass">)
            n182 = call "纳清叶绿素a_量程写入.vi"("数值"=w341, "MB session in"=w342) -> ()  [unwired: 8 in, 2 out]
            n183 = call "Add State to Queue.vi"("State(s) In (\"\")"=w343) -> ("States Out"=w345:string)  [unwired: 14 in]
          }
          event "校准启动": Value Change {
            n184 = event-data() -> ()  [unwired: 1 in, 6 out]
            n185 = global read "纳清过程全局变量.vi" "叶绿素a测试值"() -> (w348:T2)
            n186 = global read "多参数全局变量.vi" "MB session in"() -> (w349:refnum<class "MB_Master.lvclass">)
            n187 = Unbundle By Name(w348) -> ("量程"=w347:u16)
            n188 = global read "多参数全局变量.vi" "校准运行状态"() -> (w351:T5)
            n189 = Bundle By Name(cluster=w351, "叶绿素a"=TRUE ("Cond")) -> (w352:T5)
            n190 = call "纳清叶绿素a_校准量程写入.vi"("数值"=w347, "MB session in"=w349) -> ("error out"=w346:errorcluster)  [unwired: 8 in, 1 out]
            n191 = global write "多参数全局变量.vi" "校准运行状态"(w352) -> ()
            n192 = call "Add State to Queue.vi"("State(s) In (\"\")"=w356, "State(s) At Back (\"\")"="init: all\nCal: Place standard solution\n Cal: Calibration process\nidle" ("State(s) In (\"\")")) -> ("States Out"=w355:string)  [unwired: 13 in]
          }
          event "校准停止": Value Change {
            n193 = event-data() -> ()  [unwired: 1 in, 6 out]
            n194 = call "Add State to Queue.vi"("State(s) In (\"\")"="init: all\nCal: Over\nidle" ("State(s) In (\"\")")) -> ("States Out"=w358:string)  [unwired: 14 in]
          }
        }
      }
    }
  }
